vi "Power Spectrum Express.vi"() -> ()   [LabVIEW 2009]
uses:
  Instance           1 30Saved   Power Spectrum Express .vi
  <vilib>/express/express analysis/Spectral/XNode/ExpressSpectralMeasurementsBlockNode.xnode
  <vilib>/express/express analysis/Spectral/Block/exnSpectralBlock spectral measurements power poly.vi
  <vilib>/express/express analysis/Spectral/Block/exnSpectralBlock spectral measurements power DDT.vi
panel:
  out "Time Domain":dynamicdata(graph)=[{"t0"=timestamp(97.5 s since 1904-01-01), "dt"=5e-05, "Y"=array[2000 elements], "attributes"=variant("NI_ChannelName"=variant(string "Sine"), "NI_ExpIsRelativeTime"=variant(bool TRUE), "NI_ExpStartTimeStamp"=variant(timestamp timestamp(3346097903.621114 s since 1904-01-01)), "NI_ExpTimeStamp"=variant(timestamp timestamp(3346098001.121114 s since 1904-01-01)), "NI_ExpXDimension"=variant(string "t"))}] caption="Sine"
  in  "Amplitude":dbl=3.0 format="%0.2f"
  in  "stop":bool
  out "Power Spectrum":dynamicdata(graph)=[{"t0"=timestamp(0 s since 1904-01-01), "dt"=10.0, "Y"=array[1000 elements], "attributes"=variant("NI_ChannelName"=variant(string "Sine (Power Spectrum)"), "NI_ExpIsRelativeTime"=variant(bool TRUE), "NI_ExpStartTimeStamp"=variant(timestamp timestamp(3346097903.621114 s since 1904-01-01)), "NI_ExpTimeStamp"=variant(timestamp timestamp(3346098001.121114 s since 1904-01-01)), "NI_ExpXDimension"=variant(string "f"), "NI_OriginalChannelName"=variant(string "Sine"))}]
  in  "Frequency":dbl=1000.0 format="%0.2f"
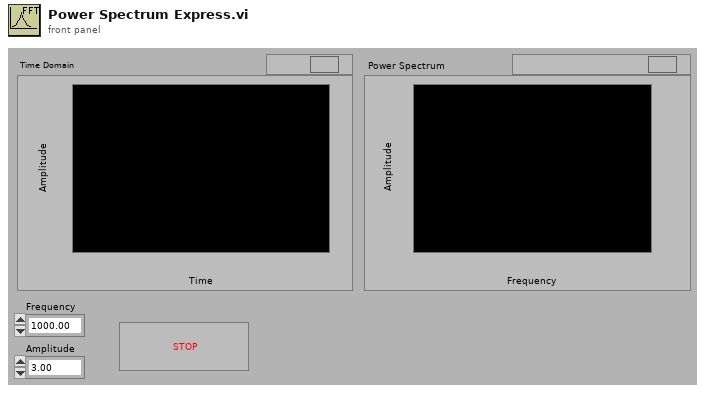
[diagram p1: front panel]
types:
  T1 = cluster{"averaging mode":u16, "weighting mode":u16, "number of averages":u32}
  T2 = cluster{"dB On (F)":bool, "unwrap phase (F)":bool, "convert to degree (F)":bool}
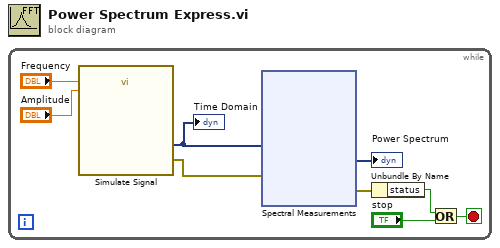
[diagram p0: block diagram]
diagram:
  n1 = while {
    stop <- w3 stop-if-true
    n2 = call "Simulate Signal"("Frequency"="Frequency", "Amplitude"="Amplitude") -> ("Sine"=w2:dynamicdata, "error out"=w8:errorcluster)  [unwired: 12 in]
    "Time Domain" <- w2
    n3 = xnode "Spectral Measurements"("Signals"=w2, "error in (no error)"=w8) -> ("Power Spectrum"=→"Power Spectrum":dynamicdata, "error out"=w6:errorcluster)
    n4 = Unbundle By Name "Unbundle By Name"(w6) -> ("status"=w5:bool)
    n5 = Or(x=w5, y="stop") -> (x .or. y?=w3:bool)
  }
